vi "onClick Callback.vi"(4 "onClick":refnum<user-event>, 5 "Event Data":cluster{"sender":refnum<k24>, "e":refnum<k24>}, 6 "Control Ref":refnum<k24>, 7 "Event Common Data":T1) -> ()   [LabVIEW 2024, in "MyEventGrid.lvclass"]
uses:
  MyEventGrid.lvclass
  D:/git/Sourcegrid-LabVIEW/dll/SourceGrid.dll
  dll/SourceGrid.dll
  MyEventGrid.lvclass/MyEventGrid.ctl
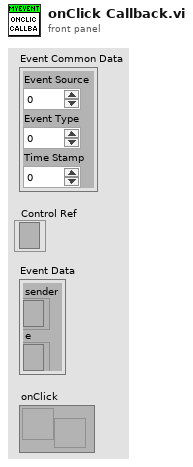
[diagram p1: front panel]
types:
  T1 = cluster{"Event Source":i32, "Event Type":u32, "Time Stamp":u32}
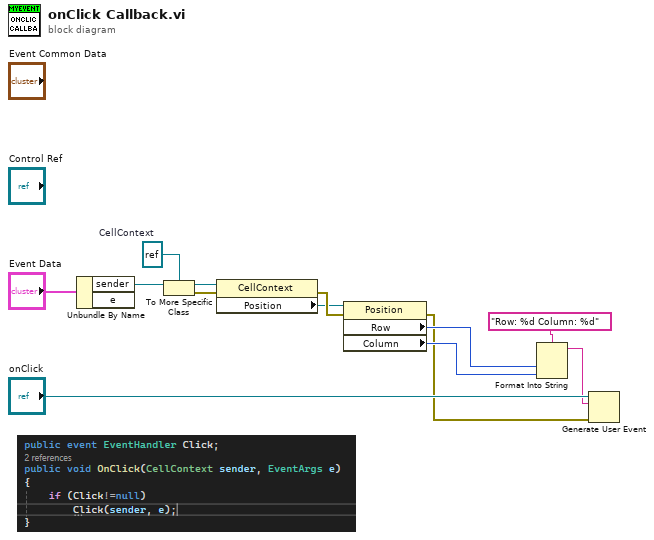
[diagram p0: block diagram]
diagram:
  w10 = refnum<k24> refnum  # CellContext
  n1 = Unbundle By Name("Event Data") -> ("sender"=w11:refnum<k24>)  [unwired: 1 out]
  n2 = To More Specific Class(target class=w10, reference=w11) -> (specific class reference=w8:refnum<k24>, error out=w9:errorcluster)  [unwired: 1 in]
  n3 = property class="CellContext"(reference=w8, error in=w9) -> (error out=w7:errorcluster, "Position"=w6:refnum<k24>)  [unwired: 1 out]
  n4 = property class="Position"(reference=w6, error in=w7) -> (error out=w2:errorcluster, "Row"=w4:i32, "Column"=w3:i32)  [unwired: 1 out]
  n5 = Format Into String(format string="Row: %d Column: %d", w4, w3) -> (resulting string=w1:string)  [unwired: 2 in, 1 out]
  n6 = Generate User Event(user event="onClick", event data cluster=w1, error in=w2) -> ()  [unwired: 1 in, 2 out]
